vi "求角度.vi"(7 "Line form(Two Point)":enum16{"Line", "Two Point"}(ring)=enum."Two Point", 9 "Point 2":cluster{"X":sgl, "Y":sgl}, 10 "Point 1":cluster{"X":sgl, "Y":sgl}, 11 "Line":T1) -> (3 "Line Data":cluster{"X":sgl, "Y":sgl, "T":sgl})   [LabVIEW 2015]
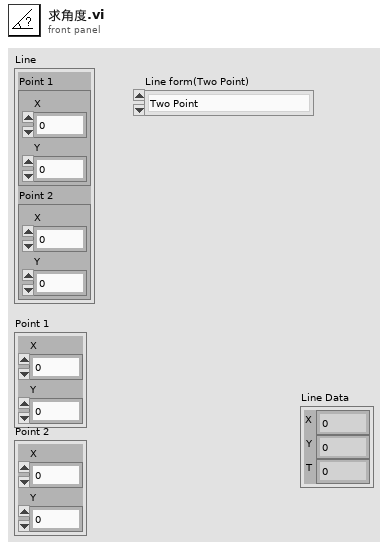
[diagram p1: front panel]
types:
  T1 = cluster{"Point 1":cluster{"X":sgl, "Y":sgl}, "Point 2":cluster{"X":sgl, "Y":sgl}}
  T2 = cluster{"center_X":dbl, "center_Y":dbl, "rotate":dbl}
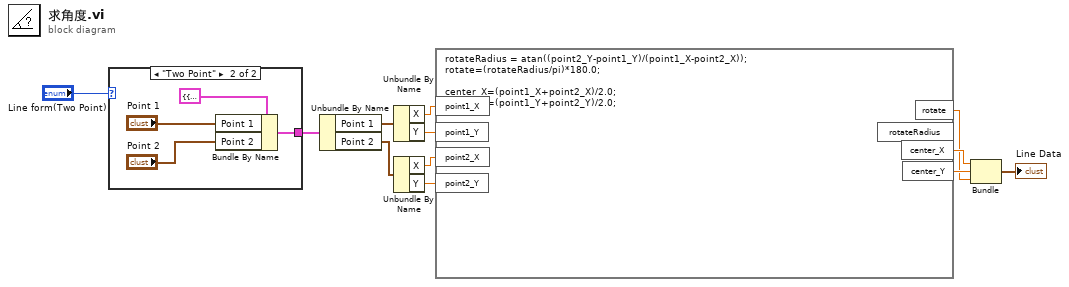
[diagram p0: block diagram]
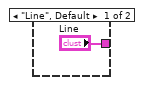
[diagram p2: hidden frame]
diagram:
  n1 = case shown="\"Two Point\"" "Line form(Two Point)" {
    tunnel: ["Line" w14] -> w9
    frame "Line", Default {
    }
    frame "Two Point" {
      n2 = Bundle By Name(cluster=T1 {"Point 1"={"X"=0.0, "Y"=0.0}, "Point 2"={"X"=0.0, "Y"=0.0}} ("Line"), "Point 1"="Point 1", "Point 2"="Point 2") -> (w14:T1)
    }
  }
  n3 = Unbundle By Name(w9) -> ("Point 1"=w11:cluster{"X":sgl, "Y":sgl}, "Point 2"=w12:cluster{"X":sgl, "Y":sgl})
  n4 = Unbundle By Name(w11) -> ("X"=w7:sgl, "Y"=w6:sgl)
  n5 = Unbundle By Name(w12) -> ("X"=w5:sgl, "Y"=w4:sgl)
  n6 = formula code="rotateRadius = atan((point2_Y-point1_Y)/(point1_X-point2_X));\nrotate=(rotateRadius/pi)*180.0;\n\ncenter_X=(point1_X+point2_X)/2.0;\ncenter_Y=(point1_Y+point2_Y)/2.0;"("point1_X"=w7, "point1_Y"=w6, "point2_X"=w5, "point2_Y"=w4) -> ("rotate"=w1:dbl, "center_X"=w3:dbl, "center_Y"=w2:dbl)  [unwired: 1 out]
  n7 = Bundle("center_X"=w3, "center_Y"=w2, "rotate"=w1) -> (→"Line Data":T2)  [unwired: 1 in]
